vi "simDataOverride.vi"(11 "CheckData in":refnum<class "CheckData.lvclass">) -> (3 "CheckData out":refnum<class "CheckData.lvclass">)   [LabVIEW 2017, in "CheckData.lvclass"]
uses:
  CheckData.lvclass
  CheckData.lvclass/CheckData.ctl
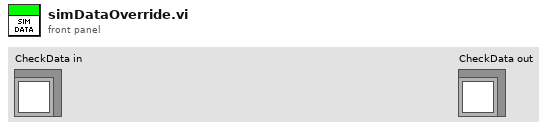
[diagram p1: front panel]
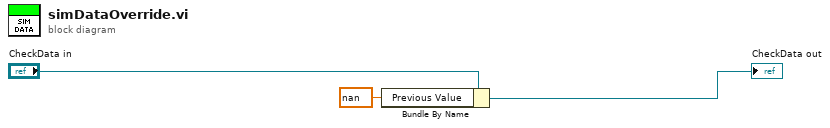
[diagram p0: block diagram]
diagram:
  n1 = Bundle By Name(cluster="CheckData in", "Previous Value"=nan) -> (→"CheckData out":refnum<class "CheckData.lvclass">)
